vi "version_check.vi"() -> ()   [LabVIEW 2017]
panel:
  in  "error in (no error)":errorcluster
  out "数组 2":errorcluster[](array[cluster])
  out "数组":u8[](array[numeric])=[38] format="%x"
  in  "Address":u32=261 format="%x"
  in  "Array":string[](array[string])=["10.3.173.20"]
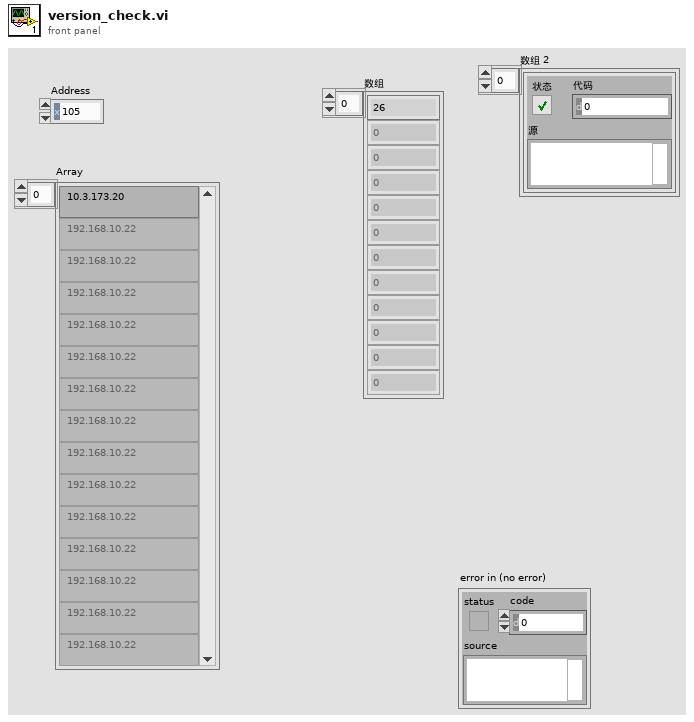
[diagram p1: front panel]
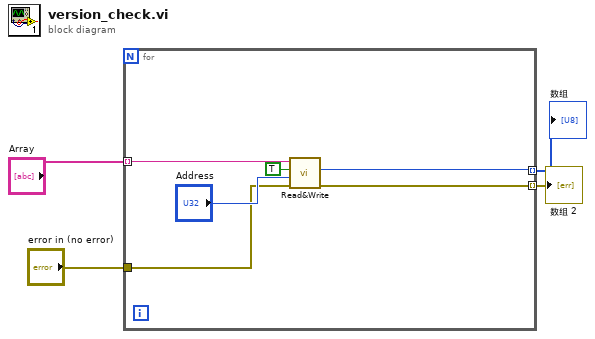
[diagram p0: block diagram]
diagram:
  n1 = for {
    tunnel: "Array" -> [w10] mode=indexing
    tunnel: [w8] -> w3 mode=indexing
    tunnel: [w7] -> w2 mode=indexing
    tunnel: "error in (no error)" -> [w5]
    n2 = call "Read&Write.vi"("error in (no error)"=w5, "Address"="Address", "Read (TRUE)"=TRUE, "address"=w10) -> ("error out"=w7:errorcluster, "Out"=w8:u8)  [unwired: 6 in]
  }
  "数组" <- w3
  "数组 2" <- w2
